vi "Gaussian Filter(3x3).vi"(6 "Input ColNum":i16, 9 "Line 3":refnum<k21>, 10 "Line 2":refnum<k21>, 11 "Line 1":refnum<k21>) -> (3 "Output":fxp<+,12,12>)   [LabVIEW 2016]
uses:
  <vilib>/rvi/DataTransferAndStorage/Container/Common/niFpgaContainerExecOnDevCompGetState.vi
  <vilib>/rvi/Emulation/niFpgaEmulationIsFPGAContextNoSignature.vi
  <vilib>/rvi/DataTransferAndStorage/Container/Common/niFpgaContainerGetUniqueNameForEmu.vi
  <vilib>/rvi/Emulation/niFpgaProcessEmulError.vi
  <vilib>/rvi/Emulation/niFpgaSctlEmulationGetInTimedLoop.vi
  <vilib>/rvi/errors/nirviReportUnexpectedCaseInternalError (U32).vi
  <vilib>/rvi/Memory/Memory_Emulation/niFpgaMemoryEmulationCacheClearOnFirstRun.vi
  <vilib>/rvi/Memory/Memory_Emulation/nirvimemoryEmulationManagerCache_MakeExclusive.vi
  <vilib>/rvi/Memory/Memory_Emulation/niFpgaMemoryEmulationValidateCache.vi
  <vilib>/rvi/Memory/Memory_Emulation/nirvimemoryEmulationManagerCache_InsertValue.vi
  <vilib>/Utility/error.llb/Clear Errors.vi
  <vilib>/rvi/Memory/Memory_Emulation/nirvimemoryEmulationManagerCache_ReleaseExclusive.vi
  <vilib>/rvi/Memory/Memory_Emulation/nirvimemoryEmulationManagerCache_GetValue.vi
  <vilib>/rvi/Memory/Memory_Emulation/nirvimemoryEmulationManagerCache_SetValue.vi
  <vilib>/rvi/Emulation/niFpgaSctlEmulationResourceMgr.vi
  <vilib>/rvi/DataTransferAndStorage/Container/XNode/niFpgaContainer.xnode
  <vilib>/rvi/Memory/Memory_Emulation/niFpgaMemoryEmulationRefIn.vi
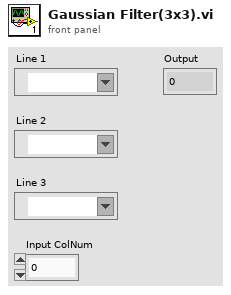
[diagram p1: front panel]
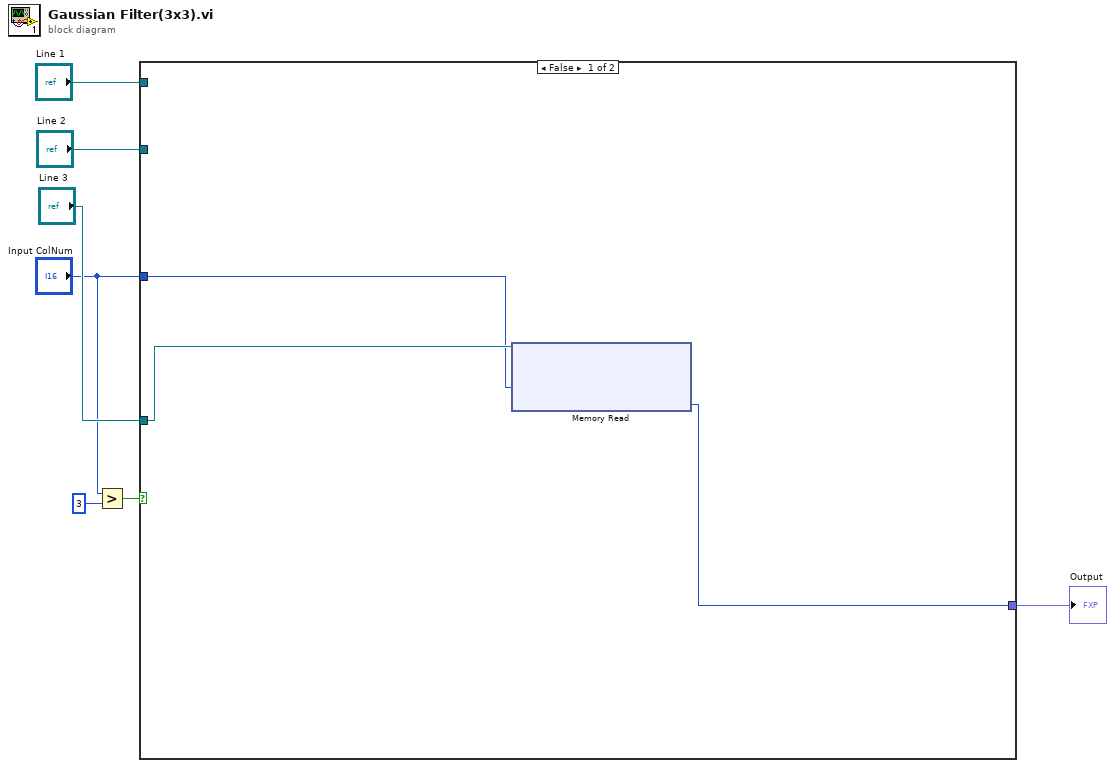
[diagram p0: block diagram]
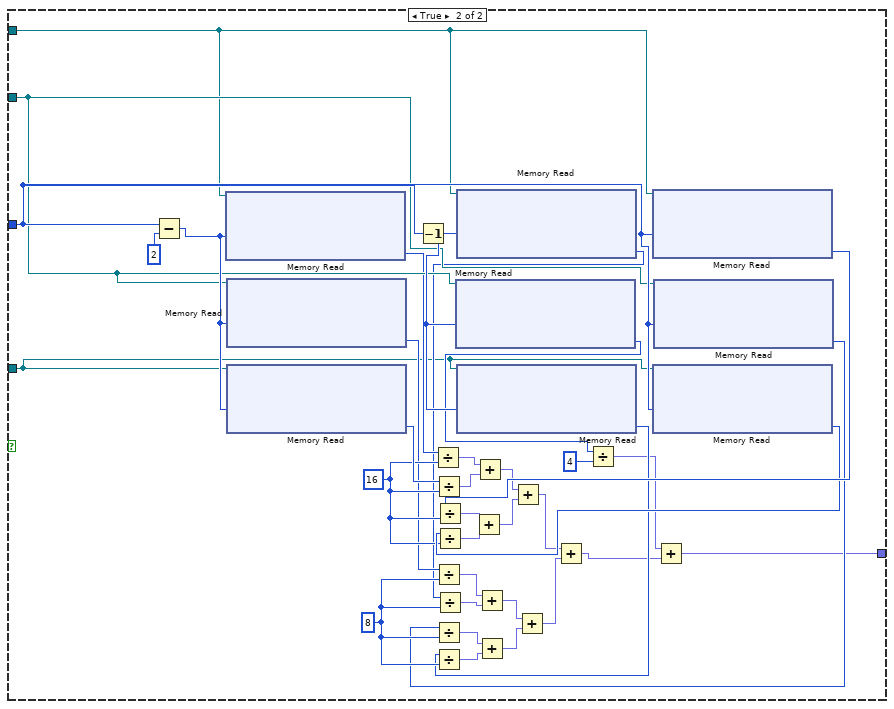
[diagram p2: hidden frame]
diagram:
  n1 = Greater?(x="Input ColNum", y=i16 3) -> (0:w3:bool)
  n2 = case shown="False" w3 {
    tunnel: "Input ColNum" -> [w9 w46]
    tunnel: "Line 2" -> [_ w43]
    tunnel: "Line 1" -> [_ w42]
    tunnel: [w8 w17] -> w5
    tunnel: "Line 3" -> [w10 w15]
    frame False {
      n3 = xnode "Memory Read"("Address"=w9, "Memory In"=w10) -> ("Data"=w8:u8)  [unwired: 1 out]
    }
    frame True {
      w28 = u8 8 ("y")
      w31 = u8 16 ("y")
      n4 = Subtract(x=w46, y=i16 2) -> (x-y=w44:i16)
      n5 = xnode "Memory Read"("Address"=w44, "Memory In"=w42) -> ("Data"=w41:u8)  [unwired: 1 out]
      n6 = xnode "Memory Read"("Address"=w44, "Memory In"=w43) -> ("Data"=w27:u8)  [unwired: 1 out]
      n7 = xnode "Memory Read"("Address"=w44, "Memory In"=w15) -> ("Data"=w40:u8)  [unwired: 1 out]
      n8 = Decrement(x=w46) -> (x-1=w45:i16)
      n9 = Divide(x=w41, y=w31) -> (x/y=w39:fxp<+,8,8>)
      n10 = Divide(x=w40, y=w31) -> (x/y=w38:fxp<+,8,8>)
      n11 = Divide(x=w27, y=w28) -> (x/y=w30:fxp<+,8,8>)
      n12 = xnode "Memory Read"("Address"=w45, "Memory In"=w43) -> ("Data"=w23:u8)  [unwired: 1 out]
      n13 = xnode "Memory Read"("Address"=w45, "Memory In"=w42) -> ("Data"=w26:u8)  [unwired: 1 out]
      n14 = Divide(x=w26, y=w28) -> (x/y=w29:fxp<+,8,8>)
      n15 = xnode "Memory Read"("Address"=w45, "Memory In"=w15) -> ("Data"=w24:u8)  [unwired: 1 out]
      n16 = Divide(x=w24, y=w28) -> (x/y=w32:fxp<+,8,8>)
      n17 = Add(x=w39, y=w38) -> (x+y=w14:fxp<+,9,9>)
      n18 = Add(x=w30, y=w29) -> (x+y=w12:fxp<+,9,9>)
      n19 = Divide(x=w23, y=u8 4) -> (x/y=w19:fxp<+,8,8>)
      n20 = xnode "Memory Read"("Address"=w46, "Memory In"=w42) -> ("Data"=w35:u8)  [unwired: 1 out]
      n21 = Divide(x=w35, y=w31) -> (x/y=w37:fxp<+,8,8>)
      n22 = xnode "Memory Read"("Address"=w46, "Memory In"=w15) -> ("Data"=w34:u8)  [unwired: 1 out]
      n23 = Divide(x=w34, y=w31) -> (x/y=w36:fxp<+,8,8>)
      n24 = Add(x=w37, y=w36) -> (x+y=w13:fxp<+,9,9>)
      n25 = Add(x=w14, y=w13) -> (x+y=w21:fxp<+,10,10>)
      n26 = xnode "Memory Read"("Address"=w46, "Memory In"=w43) -> ("Data"=w25:u8)  [unwired: 1 out]
      n27 = Divide(x=w25, y=w28) -> (x/y=w33:fxp<+,8,8>)
      n28 = Add(x=w33, y=w32) -> (x+y=w11:fxp<+,9,9>)
      n29 = Add(x=w12, y=w11) -> (x+y=w20:fxp<+,10,10>)
      n30 = Add(x=w21, y=w20) -> (x+y=w18:fxp<+,11,11>)
      n31 = Add(x=w19, y=w18) -> (x+y=w17:fxp<+,12,12>)
    }
  }
  "Output" <- w5
